vi "Case Structure.vi"() -> ()   [LabVIEW 2020]
uses:
  <vilib>/Utility/file.llb/Write Delimited Spreadsheet (DBL).vi
panel:
  in  "Numeric - I32":i32
  in  "Enum":enum16{"Meters", "Miles", "Kilometers", "Yards"}(ring)
  in  "error in (no error)":errorcluster
  in  "String":string
  in  "Boolean":bool
  in  "Numeric - Double":dbl
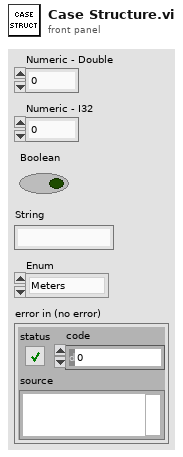
[diagram p1: front panel]
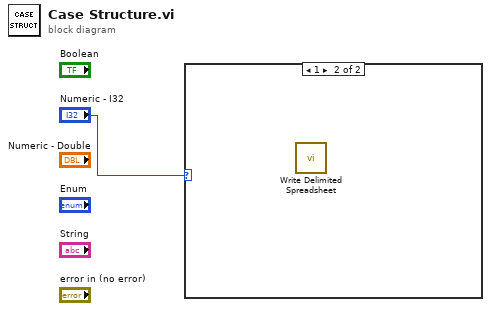
[diagram p0: block diagram]
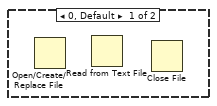
[diagram p2: hidden frame]
diagram:
  n1 = case shown="1" "Numeric - I32" {
    frame 0, Default {
      n2 = Open/Create/Replace File() -> ()  [unwired: 6 in, 3 out]
      n3 = Read from Text File() -> ()  [unwired: 4 in, 4 out]
      n4 = Close File() -> ()  [unwired: 2 in, 2 out]
    }
    frame 1 {
      n5 = call-poly <vilib>:"Write Delimited Spreadsheet.vi"() -> ()  [unwired: 14 in, 2 out]
    }
  }
